vi "create.OrderExecutedAtPriceSize.vi"(8 "error in (no error)":errorcluster, 10 "OrderExecutedAtPriceSize.Parameters":T1={"Time Offset"=447000, "Order Id"="ORID0001", "Executed Quantity"=20000, "Execution Id"="AAPL", "Remaining Quantity"=20000, "Price"=0.905}, 11 "OrderExecutedAtPriceSize in":refnum<class "OrderExecutedAtPriceSize.lvclass">) -> (0 "error out":errorcluster, 3 "OrderExecutedAtPriceSize out":refnum<class "OrderExecutedAtPriceSize.lvclass">)   [LabVIEW 2022 SP3, in "OrderExecutedAtPriceSize.lvclass"]
uses:
  OrderExecutedAtPriceSize.lvclass
  OrderExecutedAtPriceSize.Parameters.ctl
  FieldSpec.ctl
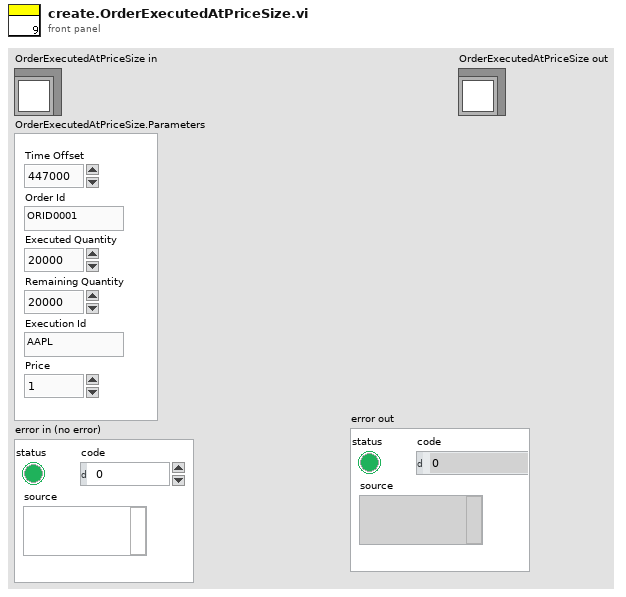
[diagram p1: front panel]
types:
  T1 = typedef "OrderExecutedAtPriceSize.lvclass/OrderExecutedAtPriceSize.Parameters.ctl" = cluster{"Time Offset":u32, "Order Id":string, "Executed Quantity":u32, "Execution Id":string, "Remaining Quantity":u32, "Price":dbl}
  T2 = typedef "FieldSpec.ctl" = cluster{"Name":string, "Offset":i32, "Length":i32, "FieldType":enum16{"Alphanumeric", "Binary", "BinaryLongPrice", "BinaryShortPrice", "BitField", "PrintableAscii", "Value"}, "FieldValue":variant}
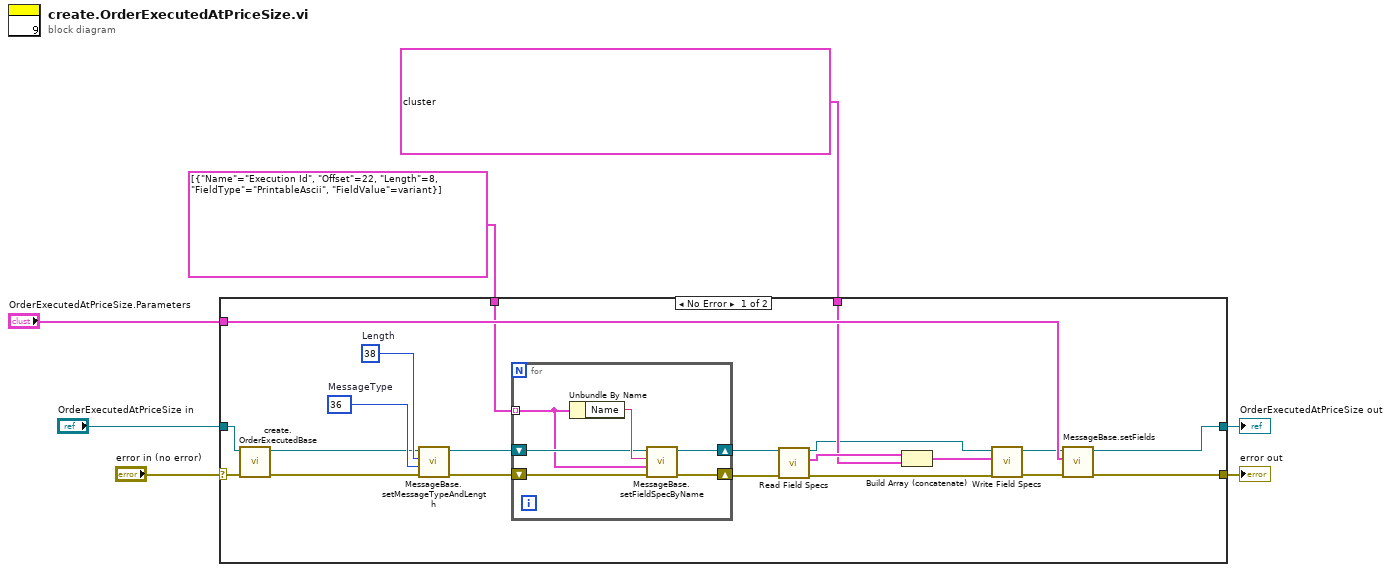
[diagram p0: block diagram]
diagram:
  n1 = case shown="No Error" "error in (no error)" {
    selector: "error in (no error)" -> [w20 w36]
    tunnel: [w24 w36] -> w6
    tunnel: [w23 w35] -> w4
    tunnel: "OrderExecutedAtPriceSize in" -> [w22 w35]
    tunnel: "OrderExecutedAtPriceSize.Parameters" -> [w21 _]
    tunnel: T2[] [{"Name"="Execution Id", "Offset"=22, "Length"=8, "FieldType"=enum."PrintableAscii", "FieldValue"=variant}] ("appended array") -> [w17 _]
    tunnel: T2[] [{"Name"="Remaining Quantity", "Offset"=18, "Length"=4, "FieldType"=enum."Binary", "FieldValue"=variant}, {"Name"="Price", "Offset"=30, "Length"=8, "FieldType"=enum."BinaryLongPrice", "FieldValue"=variant}] ("appended array") -> [w11 _]
    frame No Error {
      w27 = u8 36  # MessageType
      w28 = u8 38  # Length
      n2 = call-dynamic "create.OrderExecutedBase.vi"("error in (no error)"=w20, "OrderExecutedBase in"=w22) -> ("error out"=w26:errorcluster, "OrderExecutedBase out"=w25:refnum<class "OrderExecutedAtPriceSize.lvclass">)  [unwired: 8 in]
      n3 = call-dynamic "MessageBase.setMessageTypeAndLength.vi"("error in (no error)"=w26, "MessageType"=w27, "Length"=w28, "MessageBase in"=w25) -> ("error out"=w19:errorcluster, "MessageBase out"=w18:refnum<class "OrderExecutedAtPriceSize.lvclass">)  [unwired: 6 in]
      n4 = for {
        tunnel: w17 -> [w31] mode=indexing
        shift-right: [w29] -> w15
        shift-left: w19 -> [w33]
        shift-right: [w30] -> w16
        shift-left: w18 -> [w32]
        n5 = Unbundle By Name(w31) -> ("Name"=w34:string)
        n6 = call-dynamic "MessageBase.setFieldSpecByName.vi"("error in (no error)"=w33, "FIeldSpec"=w31, "Field.Name"=w34, "MessageBase in"=w32) -> ("error out"=w29:errorcluster, "MessageBase out"=w30:refnum<class "OrderExecutedAtPriceSize.lvclass">)  [unwired: 6 in]
      }
      n7 = call-dynamic "Read Field Specs.vi"("error in (no error)"=w15, "MessageBase in"=w16) -> ("error out"=w9:errorcluster, "Field Specs"=w12:T2[], "MessageBase out"=w8:refnum<class "OrderExecutedAtPriceSize.lvclass">)  [unwired: 7 in]
      n8 = Build Array (concatenate)(w12, w11) -> (w10:T2[])
      n9 = call-dynamic "Write Field Specs.vi"("error in (no error)"=w9, "Field Specs"=w10, "MessageBase in"=w8) -> ("error out"=w14:errorcluster, "MessageBase out"=w13:refnum<class "OrderExecutedAtPriceSize.lvclass">)  [unwired: 7 in]
      n10 = call-dynamic "MessageBase.setFields.vi"("error in (no error)"=w14, "Cluster (dup)"=w21, "MessageBase in"=w13) -> ("error out"=w24:errorcluster, "MessageBase out"=w23:refnum<class "OrderExecutedAtPriceSize.lvclass">)  [unwired: 7 in]
    }
    frame Error {
    }
  }
  "error out" <- w6
  "OrderExecutedAtPriceSize out" <- w4
